vi "Field Draw Path.vi"(0 "Pontos Smooth":dbl[][](array[numeric]), 4 "Lado":enum16{"Esquerdo", "Direito"}(ring) caption="Enum", 6 "Draw Targets?":T2, 8 "Scale mm/pixel":dbl, 9 "Offset":T3, 10 "Pontos":dbl[][](array[numeric]), 11 "picture in":picture) -> (2 "picture out":picture)   [LabVIEW 2016]
uses:
  <vilib>/Utility/miscctls.llb/LVBoundsTypeDef.ctl
  DrawTargets.ctl
panel:
  in  "pen 2":T1={"Width"=3, "Style"=enum."Solid"}
  in  "pen":T1={"Width"=3, "Style"=enum."Solid"}
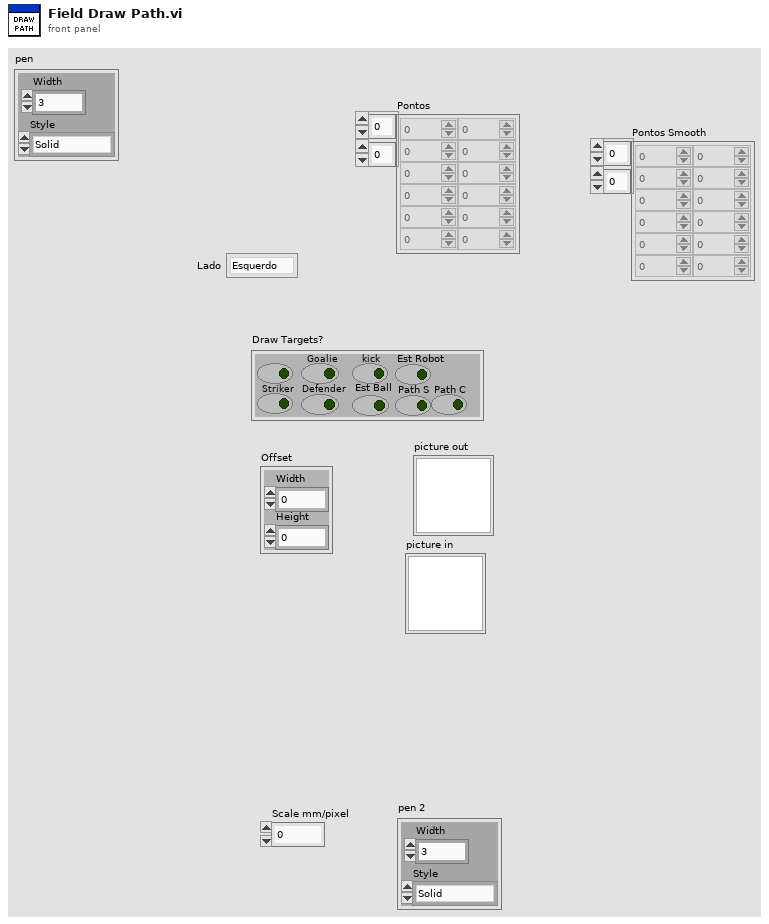
[diagram p1: front panel]
types:
  T1 = cluster{"Width":u16, "Style":enum32{"Solid", "Dash", "Dot", "DashDot", "DashDotDot"}}
  T2 = typedef "DrawTargets.ctl" = cluster{"Attacker":bool, "Striker":bool, "Goalie":bool, "Defender":bool, "kick":bool, "Est Ball":bool, "Est Robot":bool, "Path S":bool, "Path C":bool}
  T3 = typedef "LVBoundsTypeDef.ctl" = cluster{"Width":u32, "Height":u32}
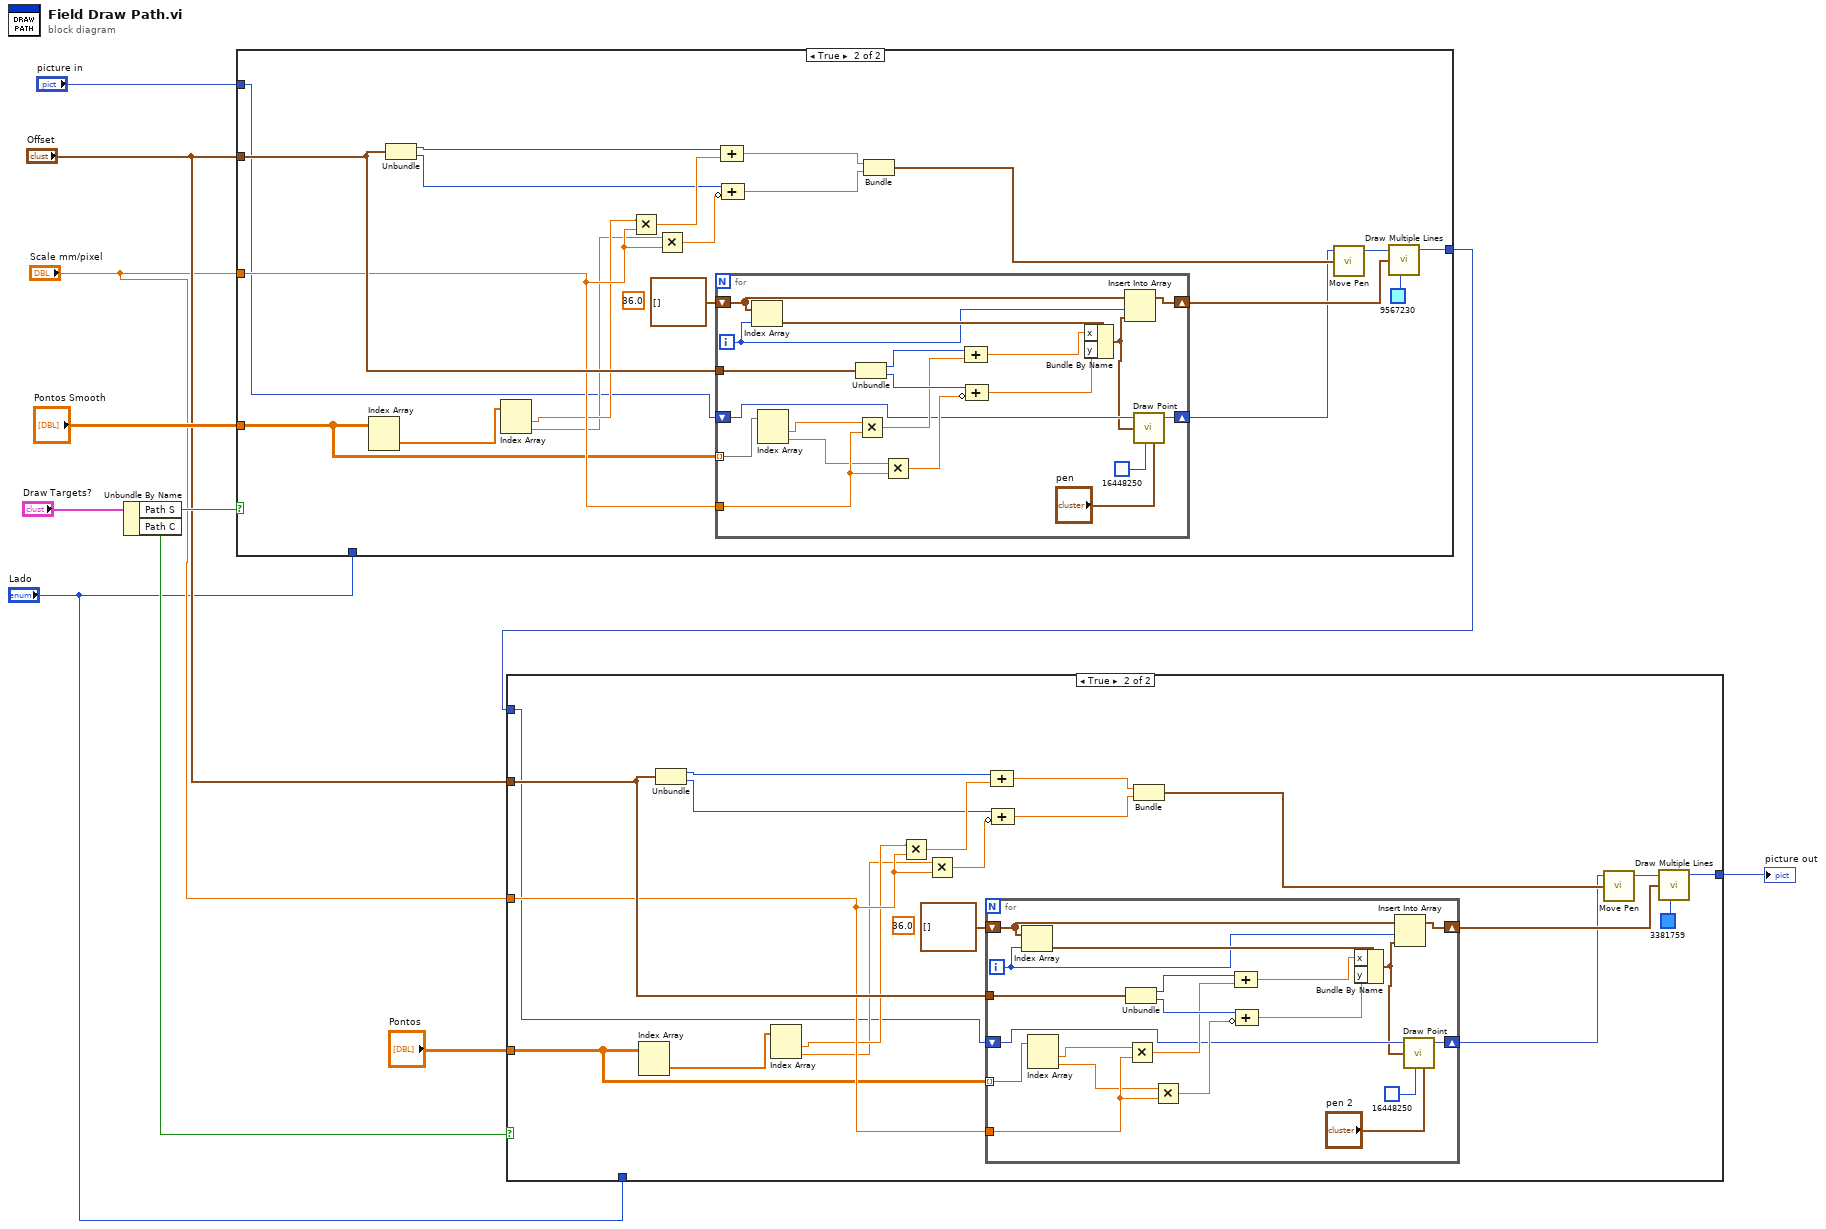
[diagram p0: block diagram]
diagram:
  n1 = Unbundle By Name("Draw Targets?") -> ("Path S"=w9:bool, "Path C"=w3:bool)
  n2 = case shown="True" w9 {
    tunnel: [w12 w13] -> w7
    tunnel: "Offset" -> [_ w25]
    tunnel: "Scale mm/pixel" -> [_ w24]
    tunnel: "picture in" -> [w12 w15]
    tunnel: "Lado" -> [_ _]
    tunnel: "Pontos Smooth" -> [_ w18]
    frame False {
    }
    frame True {
      (unwired) sgl 36.0 ("radius")
      n3 = Index Array(array=w18) -> (element=w21:dbl[])  [unwired: 2 in]
      n4 = Unbundle(w25) -> ("Width"=w32:u32, "Height"=w29:u32)
      n5 = Index Array(array=w21) -> (element #1=w20:dbl, element #2=w19:dbl)  [unwired: 2 in]
      n6 = Multiply(x=w20, y=w24) -> (x*y=w31:dbl)
      n7 = Multiply(x=w19, y=w24) -> (x*y=w28:dbl)
      n8 = for {
        tunnel: w25 -> [w50]
        tunnel: w24 -> [w49]
        tunnel: w18 -> [w46] mode=indexing
        shift-right: [w38] -> w16
        shift-left: cluster{"x":i16, "y":i16}[] [] ("line endpoints") -> [w39]
        shift-right: [w36] -> w14
        shift-left: w15 -> [w37]
        i -> [w40]
        n9 = Index Array(array=w39, index=w40) -> (element=w41:cluster{"x":i16, "y":i16})
        n10 = Index Array(array=w46) -> (element #1=w45:dbl, element #2=w44:dbl)  [unwired: 2 in]
        n11 = Unbundle(w50) -> ("Width"=w52:u32, "Height"=w51:u32)
        n12 = Multiply(x=w45, y=w49) -> (x*y=w48:dbl)
        n13 = Multiply(x=w44, y=w49) -> (x*y=w47:dbl)
        n14 = Compound Arithmetic op=ADD(w52, w48) -> (w43:dbl)
        n15 = Compound Arithmetic op=ADD(w51, invert w47) -> (w42:dbl)
        n16 = Bundle By Name(cluster=w41, "x"=w43, "y"=w42) -> (w34:cluster{"x":i16, "y":i16})
        n17 = Insert Into Array(array=w39, index=w40, new element=w34) -> (w38:cluster{"x":i16, "y":i16}[])
        n18 = call <vilib>:"Draw Point.vi"("picture"=w37, "point(x,y)"=w34, "color(black)"=u32 16448250, "pen"="pen") -> ("new picture"=w36:picture)  [unwired: 5 in]
      }
      n19 = Compound Arithmetic op=ADD(w32, w31) -> (w30:dbl)
      n20 = Compound Arithmetic op=ADD(w29, invert w28) -> (w27:dbl)
      n21 = Bundle(w30, w27) -> (w22:cluster{dbl, dbl})  [unwired: 1 in]
      n22 = call <vilib>:"Move Pen.vi"("new position"=w22, "picture"=w14) -> ("new picture"=w26:picture)  [unwired: 3 in]
      n23 = call <vilib>:"Draw Multiple Lines.vi"("picture"=w26, "line endpoints"=w16, "color(black)"=u32 9567230) -> ("new picture"=w13:picture)  [unwired: 6 in]
    }
  }
  n24 = case shown="True" w3 {
    tunnel: [w53 w54] -> w1
    tunnel: "Offset" -> [_ w66]
    tunnel: "Scale mm/pixel" -> [_ w65]
    tunnel: w7 -> [w53 w56]
    tunnel: "Lado" -> [_ _]
    tunnel: "Pontos" -> [_ w59]
    frame False {
    }
    frame True {
      (unwired) sgl 36.0 ("radius")
      n25 = Index Array(array=w59) -> (element=w62:dbl[])  [unwired: 2 in]
      n26 = Unbundle(w66) -> ("Width"=w73:u32, "Height"=w70:u32)
      n27 = Index Array(array=w62) -> (element #1=w61:dbl, element #2=w60:dbl)  [unwired: 2 in]
      n28 = Multiply(x=w61, y=w65) -> (x*y=w72:dbl)
      n29 = Multiply(x=w60, y=w65) -> (x*y=w69:dbl)
      n30 = for {
        tunnel: w66 -> [w91]
        tunnel: w65 -> [w90]
        tunnel: w59 -> [w87] mode=indexing
        shift-right: [w79] -> w57
        shift-left: cluster{"x":i16, "y":i16}[] [] ("line endpoints") -> [w80]
        shift-right: [w77] -> w55
        shift-left: w56 -> [w78]
        i -> [w81]
        n31 = Index Array(array=w80, index=w81) -> (element=w82:cluster{"x":i16, "y":i16})
        n32 = Index Array(array=w87) -> (element #1=w86:dbl, element #2=w85:dbl)  [unwired: 2 in]
        n33 = Unbundle(w91) -> ("Width"=w93:u32, "Height"=w92:u32)
        n34 = Multiply(x=w86, y=w90) -> (x*y=w89:dbl)
        n35 = Multiply(x=w85, y=w90) -> (x*y=w88:dbl)
        n36 = Compound Arithmetic op=ADD(w93, w89) -> (w84:dbl)
        n37 = Compound Arithmetic op=ADD(w92, invert w88) -> (w83:dbl)
        n38 = Bundle By Name(cluster=w82, "x"=w84, "y"=w83) -> (w75:cluster{"x":i16, "y":i16})
        n39 = Insert Into Array(array=w80, index=w81, new element=w75) -> (w79:cluster{"x":i16, "y":i16}[])
        n40 = call <vilib>:"Draw Point.vi"("picture"=w78, "point(x,y)"=w75, "color(black)"=u32 16448250, "pen"="pen 2") -> ("new picture"=w77:picture)  [unwired: 5 in]
      }
      n41 = Compound Arithmetic op=ADD(w73, w72) -> (w71:dbl)
      n42 = Compound Arithmetic op=ADD(w70, invert w69) -> (w68:dbl)
      n43 = Bundle(w71, w68) -> (w63:cluster{dbl, dbl})  [unwired: 1 in]
      n44 = call <vilib>:"Move Pen.vi"("new position"=w63, "picture"=w55) -> ("new picture"=w67:picture)  [unwired: 3 in]
      n45 = call <vilib>:"Draw Multiple Lines.vi"("picture"=w67, "line endpoints"=w57, "color(black)"=u32 3381759) -> ("new picture"=w54:picture)  [unwired: 6 in]
    }
  }
  "picture out" <- w1
